vi "List Objects Recursive.vi"(6 "Remaining objs":u32, 7 "marker":string, 8 "error in (no error)":errorcluster, 9 "Prefix":string, 10 "Delimiter":string, 11 "Bucket in":refnum<class "Bucket.lvclass">) -> (0 "error out":errorcluster, 1 "CommonPrefixes":T1[](array[typedef]), 2 "Objects":T2[](array[typedef]), 3 "Bucket out":refnum<class "Bucket.lvclass">)   [LabVIEW 2015, in "NI_AWS_S3.lvlib" / "Bucket.lvclass"]
uses:
  Bucket.lvclass
  Object/Object.lvclass
  Object Content.ctl
  Storage Class.ctl
  Owner.ctl
  Common Prefix.ctl
  Core/HTTP Request/Request Options.ctl
  Core/HTTP Request/Name Value Pair.ctl
  Core/HTTP Request/Region handling.ctl
  Core/HTTP Request/URL formatting.ctl
  Bucket.lvclass/Bucket.ctl
  Read Name.vi
  Core/HTTP Request/HTTP Request.lvclass
  NI_AWS_S3.lvlib
panel:
  out "Objects":refnum<class "Object.lvclass">[](array[class])
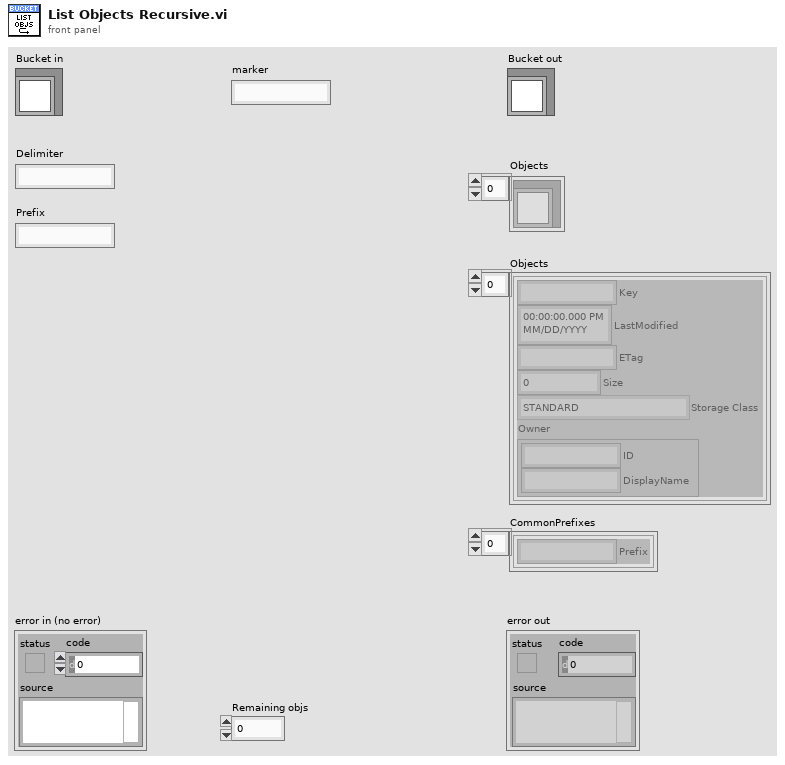
[diagram p1: front panel]
types:
  T1 = typedef "NI_AWS_S3.lvlib/Common Prefix.ctl" = cluster{"Prefix":string}
  T2 = typedef "NI_AWS_S3.lvlib/Object Content.ctl" = cluster{"Key":string, "LastModified":timestamp, "ETag":string, "Size":u64, "Storage Class":T3, "Owner":T4}
  T3 = typedef "NI_AWS_S3.lvlib/Storage Class.ctl" = enum16{"STANDARD", "REDUCED_REDUNDANCY"}
  T4 = typedef "NI_AWS_S3.lvlib/Owner.ctl" = cluster{"ID":string, "DisplayName":string}
  T5 = typedef "NI_AWS_Core.lvlib/HTTP Request.lvclass/Name Value Pair.ctl" = cluster{"name":string, "value":string}
  T6 = typedef "NI_AWS_Core.lvlib/HTTP Request.lvclass/Region handling.ctl" = enum16{"use region everywhere", "use region (authentication only)", "use region (URL only)", "ignore region everwhere"}
  T7 = typedef "NI_AWS_Core.lvlib/HTTP Request.lvclass/Request Options.ctl" = cluster{"request headers":T5[], "request parameters":T5[], "request body":string, "region handling":T6, "URL formatting":T8}
  T8 = typedef "NI_AWS_Core.lvlib/HTTP Request.lvclass/URL formatting.ctl" = enum16{"region-", "region."}
  T9 = typedef "NI_AWS_Core.lvlib/HTTP Request.lvclass/Response.ctl" = cluster{"Headers":string, "Body":string}
  T10 = typedef "NI_AWS_S3.lvlib/List Objects Result.ctl" = cluster{"Name":string, "Prefix":string, "Marker":string, "MaxKeys":u16, "IsTruncated?":bool, "Contents":T2[], "CommonPrefixes":T1[]}
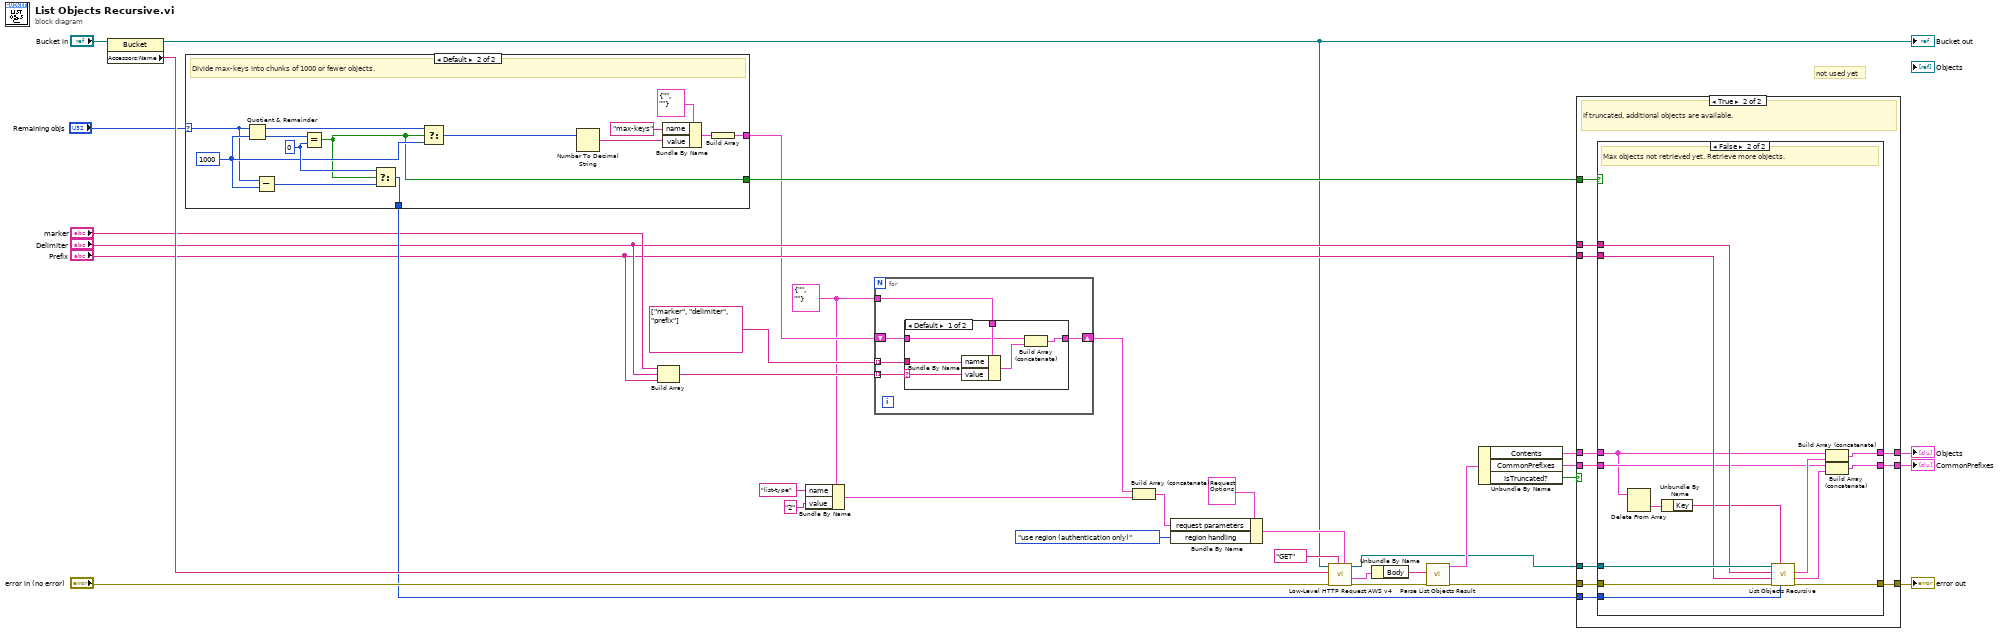
[diagram p0: block diagram]
diagram:
  w6 = T5 {"name"="", "value"=""} ("Name Value Pair")
  # "not used yet"
  n1 = property class="Bucket"(reference="Bucket in") -> (reference out=w2:refnum<class "Bucket.lvclass">, "Accessors:Name"=w32:string)  [unwired: 1 in, 1 out]
  "Bucket out" <- w2
  n2 = case shown="Default" "Remaining objs" {
    selector: "Remaining objs" -> [w36 w40]
    tunnel: [w36 w43] -> w14
    tunnel: [_ w39] -> w13
    tunnel: [_ w37] -> w9
    frame 0 {
      # "Do not specify max-keys if zero. Retrieve all objects."
    }
    frame Default {
      w44 = u32 0
      w42 = u32 1000 ("y")
      # "Divide max-keys into chunks of 1000 or fewer objects."
      n3 = Quotient & Remainder(x=w40, y=w42) -> (x-y*floor(x/y)=w45:u32, floor(x/y)=w47:u32)
      n4 = Subtract(x=w40, y=w42) -> (x-y=w41:u32)
      n5 = Equal?(x=w47, y=w44) -> (x = y?=w39:bool)
      n6 = Select(t=w44, s=w39, f=w41) -> (s? t:f=w43:u32)
      n7 = Select(t=w45, s=w39, f=w42) -> (s? t:f=w46:u32)
      n8 = Number To Decimal String(number=w46) -> (decimal integer string=w48:string)  [unwired: 1 in]
      n9 = Bundle By Name(cluster=T5 {"name"="", "value"=""} ("Name Value Pair"), "name"="max-keys", "value"=w48) -> (w38:T5)
      n10 = Build Array(w38) -> (w37:T5[])
    }
  }
  n11 = Build Array("marker", "Delimiter", "Prefix") -> (w8:string[])
  n12 = Bundle By Name(cluster=w6, "name"="list-type", "value"="2") -> (w28:T5)
  n13 = for {
    shift-right: [w55] -> w17
    shift-left: w9 -> [w54]
    tunnel: w8 -> [w53] mode=indexing
    tunnel: string[] ["marker", "delimiter", "prefix"] -> [w52] mode=indexing
    tunnel: w6 -> [w51]
    n14 = case shown="Default" w53 {
      selector: w53 -> [w60 _]
      tunnel: [w57 w62] -> w55
      tunnel: w51 -> [w61 _]
      tunnel: w54 -> [w59 w62]
      tunnel: w52 -> [w56 _]
      frame Default {
        n15 = Bundle By Name(cluster=w61, "name"=w56, "value"=w60) -> (w58:T5)
        n16 = Build Array (concatenate)(w59, w58) -> (w57:T5[])
      }
      frame "" {
      }
    }
  }
  n17 = Build Array (concatenate)(w17, w28) -> (w27:T5[])
  n18 = Bundle By Name(cluster=T7 {"request headers"=[], "request parameters"=[], "request body"="", "region handling"=enum."use region everywhere", "URL formatting"=enum."region."} ("Request Options"), "request parameters"=w27, "region handling"=Region_handling."use region (authentication only)") -> (w3:T7)
  n19 = call "Low-Level HTTP Request AWS v4.vi"("Request Options"=w3, "HTTP-Verb"="GET", "error in (no error)"="error in (no error)", "URL Prefix"=w32, "AWS Core in"=w2) -> ("error out"=w25:errorcluster, "Response"=w5:T9, "AWS Core out"=w1:refnum<class "Bucket.lvclass">)  [unwired: 3 in, 1 out]
  n20 = Unbundle By Name(w5) -> ("Body"=w26:string)
  n21 = call "Parse List Objects Result.vi"("error in (no error)"=w25, "Response body"=w26) -> ("error out"=w22:errorcluster, "List Objects Result"=w24:T10)  [unwired: 8 in]
  n22 = Unbundle By Name(w24) -> ("Contents"=w20:T2[], "CommonPrefixes"=w19:T1[], "IsTruncated?"=w23:bool)
  n23 = case shown="True" w23 {
    tunnel: w1 -> [_ w76]
    tunnel: w22 -> [w63 w75]
    tunnel: [w63 w74] -> w21
    tunnel: "Delimiter" -> [_ w73]
    tunnel: "Prefix" -> [_ w72]
    tunnel: w20 -> [w65 w68]
    tunnel: [w65 w71] -> w16
    tunnel: w19 -> [w64 w70]
    tunnel: [w64 w69] -> w18
    tunnel: w14 -> [_ w67]
    tunnel: w13 -> [_ w66]
    frame False {
      # "Data was not truncated. No more objects left."
    }
    frame True {
      # "If truncated, additional objects are available."
      n24 = case shown="False" w66 {
        tunnel: w76 -> [_ w93]
        tunnel: w75 -> [w77 w92]
        tunnel: [w77 w91] -> w74
        tunnel: w73 -> [_ w90]
        tunnel: w72 -> [_ w89]
        tunnel: [w79 w87] -> w71
        tunnel: w70 -> [w78 w86]
        tunnel: [w78 w84] -> w69
        tunnel: w68 -> [w79 w83]
        tunnel: w67 -> [_ w80]
        frame True {
          # "More objects are available, but max objects retrieved. Return from recursion."
        }
        frame False {
          # "Max objects not retrieved yet. Retrieve more objects."
          n25 = Delete From Array(array=w83) -> (deleted portion=w82:T2)  [unwired: 2 in, 1 out]
          n26 = Unbundle By Name(w82) -> ("Key"=w81:string)
          n27 = call "List Objects Recursive.vi"("Remaining objs"=w80, "marker"=w81, "error in (no error)"=w92, "Prefix"=w89, "Delimiter"=w90, "Bucket in"=w93) -> ("error out"=w91:errorcluster, "CommonPrefixes"=w85:T1[], "Objects"=w88:T2[])  [unwired: 2 in, 1 out]
          n28 = Build Array (concatenate)(w83, w88) -> (w87:T2[])
          n29 = Build Array (concatenate)(w86, w85) -> (w84:T1[])
        }
      }
    }
  }
  "error out" <- w21
  "Objects" <- w16
  "CommonPrefixes" <- w18
